vi "Get Mouse Location (Connections).vi"(10 "Event Coord":T1, 11 "Connections Reference":refnum<vi>) -> (1 "Element Reference":refnum<vi>, 2 "Type":enum16{"Source", "Destination", "Neither"}(ring), 3 "Array Index":i32)   [LabVIEW 2017, in "Routing and Faulting System Explorer.lvlib"]
uses:
  Routing and Faulting System Explorer.lvlib
  <vilib>/Utility/miscctls.llb/LVPoint32TypeDef.ctl
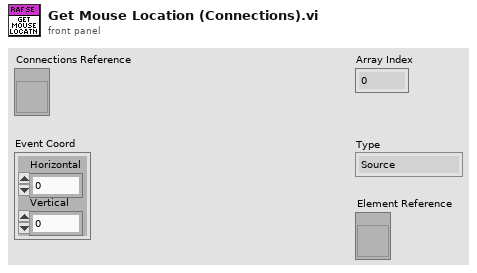
[diagram p1: front panel]
types:
  T1 = typedef "LVPoint32TypeDef.ctl" = cluster{"Horizontal":i32, "Vertical":i32}
  T2 = typedef "Routing and Faulting System Explorer.lvlib/Connection Row.ctl" = cluster{"Source":string, "Destination":string, "Edit":bool, "Remove":bool}
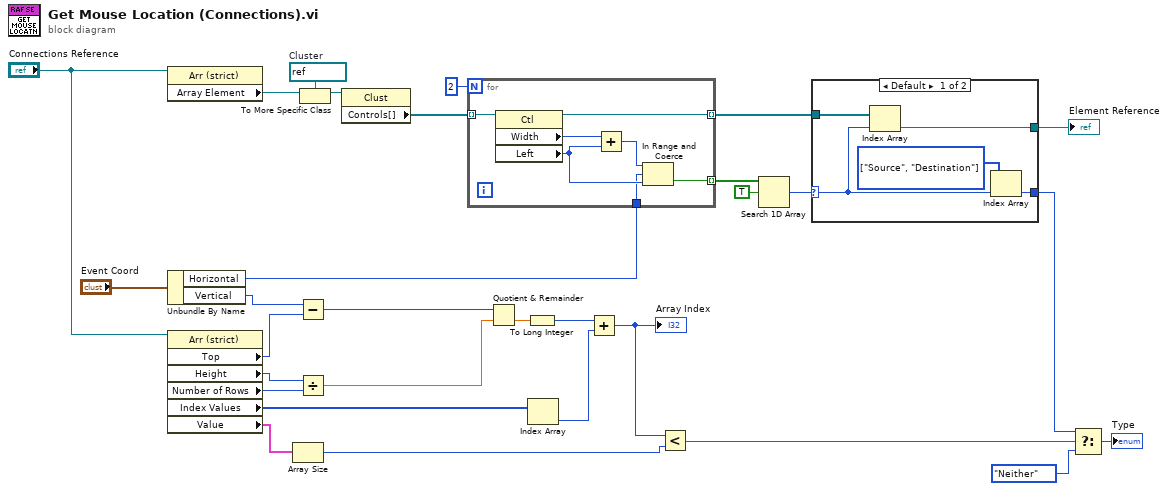
[diagram p0: block diagram]
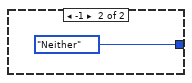
[diagram p2: hidden frame]
diagram:
  w30 = refnum<vi> refnum  # Cluster
  n1 = property on="Property Node" class="Arr (strict)"(reference="Connections Reference") -> ("Array Element"=w28:refnum<vi>)  [unwired: 1 in, 2 out]
  n2 = Unbundle By Name("Event Coord") -> ("Horizontal"=w13:i32, "Vertical"=w19:i32)
  n3 = property on="Property Node" class="Arr (strict)"(reference="Connections Reference") -> ("Top"=w20:i32, "Height"=w21:u32, "Number of Rows"=w23:u32, "Index Values"=w17:u32[], "Value"=w7:T2[])  [unwired: 1 in, 2 out]
  n4 = Array Size(array=w7) -> (size(s)=w5:i32)
  n5 = Subtract(x=w19, y=w20) -> (x-y=w27:i32)
  n6 = Divide(x=w21, y=w23) -> (x/y=w26:dbl)
  n7 = To More Specific Class(target class=w30, reference=w28) -> (specific class reference=w29:refnum<vi>)  [unwired: 1 in, 1 out]
  n8 = property class="Clust"(reference=w29) -> ("Controls[]"=w15:refnum<vi>[])  [unwired: 1 in, 2 out]
  n9 = for {
    N: 2 -> [_]
    tunnel: [w35] -> w12 mode=indexing
    tunnel: w15 -> [w33] mode=indexing
    tunnel: w13 -> [w32]
    tunnel: [w31] -> w9 mode=indexing
    n10 = property on="Property Node" class="Ctl"(reference=w33) -> (reference out=w31:refnum<vi>, "Width"=w34:u32, "Left"=w36:i32)  [unwired: 1 in, 1 out]
    n11 = Add(x=w34, y=w36) -> (x+y=w37:u32)
    n12 = In Range and Coerce(upper limit=w37, x=w32, lower limit=w36) -> (In Range?=w35:bool)  [unwired: 1 out]
  }
  n13 = Quotient & Remainder(x=w27, y=w26) -> (floor(x/y)=w25:dbl)  [unwired: 1 out]
  n14 = To Long Integer(number=w25) -> (32bit integer=w24:i32)
  n15 = Index Array(array=w17) -> (element=w16:u32)  [unwired: 1 in]
  n16 = Add(x=w24, y=w16) -> (x+y=w6:u32)
  "Array Index" <- w6
  n17 = Less?(x=w6, y=w5) -> (x < y?=w4:bool)
  n18 = Search 1D Array(1D array=w12, element=TRUE) -> (index of element=w10:i32)  [unwired: 1 in]
  n19 = case shown="Default" w10 {
    selector: w10 -> [w38 _]
    tunnel: w9 -> [w42 _]
    tunnel: [w41 _] -> w8
    tunnel: [w39 enum16{"Source", "Destination", "Neither"}."Neither" ("type")] -> w3
    frame Default {
      w40 = enum16{"Source", "Destination", "Neither"}[] [enum."Source", enum."Destination"] items=["Source", "Destination", "Neither"]
      n20 = Index Array(array=w42, index=w38) -> (element=w41:refnum<vi>)
      n21 = Index Array(array=w40, index=w38) -> (element=w39:enum16{"Source", "Destination", "Neither"})
    }
    frame -1 {
    }
  }
  "Element Reference" <- w8
  n22 = Select(t=w3, s=w4, f=enum16{"Source", "Destination", "Neither"}."Neither" ("type")) -> (s? t:f=→"Type":enum16{"Source", "Destination", "Neither"})
